vi "Copy to Matching Items.vi"(9 "Front Panel Controls":T1, 11 "VI Data":T2[](array[typedef])) -> (3 "VI Data out":T2[](array[typedef]))   [LabVIEW 2023, in "VI Properties Editor.lvlib"]
doc: "Copies current VI properties to all VIs whose name matches the one currently being edited."
uses:
  VI Properties Editor.lvlib
  <vilib>/picture/picture.llb/imagedata.ctl
  CTLs/VI Data.ctl
  CTLs/VI Properties.ctl
  CTLs/Control Properties.ctl
  CTLs/Main Front Panel Controls.ctl
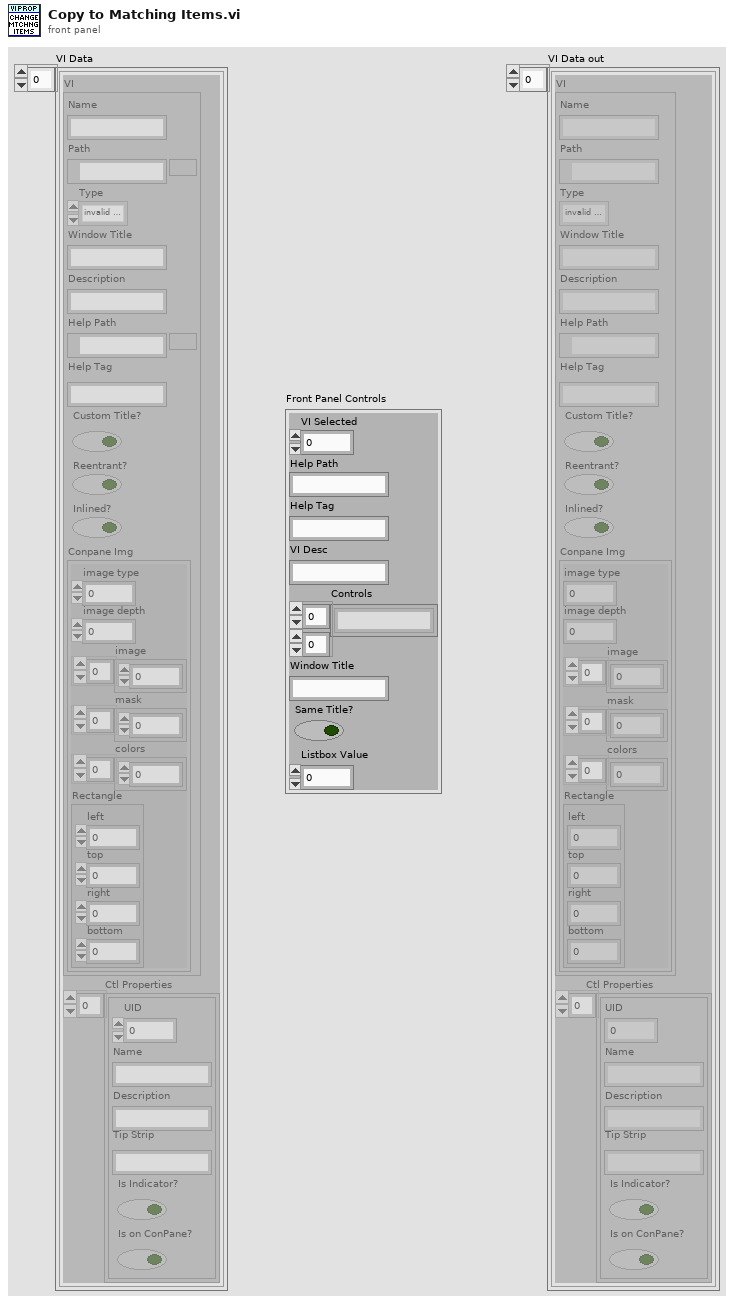
[diagram p1: front panel]
types:
  T1 = typedef "VI Properties Editor.lvlib/Main Front Panel Controls.ctl" = cluster{"VI Selected":i32, "Help Path":string, "Help Tag":string, "VI Desc":string, "Controls":string[][], "Window Title":string, "Same Title?":bool, "Listbox Value":i32}
  T2 = typedef "VI Properties Editor.lvlib/VI Data.ctl" = cluster{"VI":T3, "Ctl Properties":T5[]}
  T3 = typedef "VI Properties Editor.lvlib/VI Properties.ctl" = cluster{"Name":string, "Path":path, "Type":enum32{"invalid VI type", "Standard VI", "Control VI", "Global VI", "Polymorphic VI", "Configuration VI", "SubSystem", "Facade VI", "Method VI", "Statechart Diagram VI"}, "Window Title":string, "Description":string, "Help Path":path, "Help Tag":string, "Custom Title?":bool, "Reentrant?":bool, "Inlined?":bool, "Conpane Img":T4}
  T4 = typedef "imagedata.ctl" = cluster{"image type":i32, "image depth":i32, "image":u8[], "mask":u8[], "colors":u32[], "Rectangle":cluster{"left":i16, "top":i16, "right":i16, "bottom":i16}}
  T5 = typedef "VI Properties Editor.lvlib/Control Properties.ctl" = cluster{"UID":i32, "Name":string, "Description":string, "Tip Strip":string, "Is Indicator?":bool, "Is on ConPane?":bool}
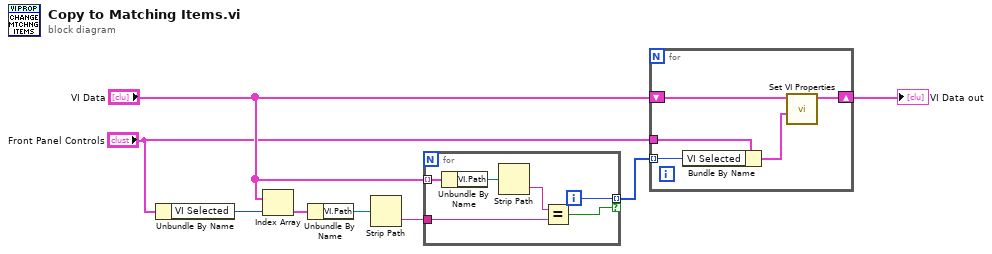
[diagram p0: block diagram]
diagram:
  n1 = Unbundle By Name("Front Panel Controls") -> ("VI Selected"=w4:i32)
  n2 = Index Array(array="VI Data", index=w4) -> (element=w6:T2)
  n3 = Unbundle By Name(w6) -> ("VI.Path"=w3:path)
  n4 = Strip Path(path=w3) -> (name=w2:string)  [unwired: 1 out]
  n5 = for {
    tunnel: "VI Data" -> [w10] mode=indexing
    tunnel: w2 -> [w14]
    tunnel: [w12] -> w7 mode=indexing if=w11
    i -> [w12]
    n6 = Unbundle By Name(w10) -> ("VI.Path"=w9:path)
    n7 = Strip Path(path=w9) -> (name=w13:string)  [unwired: 1 out]
    n8 = Equal?(x=w13, y=w14) -> (x = y?=w11:bool)
  }
  n9 = for {
    tunnel: w7 -> [w16] mode=indexing
    shift-right: [w15] -> w8
    shift-left: "VI Data" -> [w19]
    tunnel: "Front Panel Controls" -> [w18]
    n10 = Bundle By Name(cluster=w18, "VI Selected"=w16) -> (w17:T1)
    n11 = call "Set VI Properties.vi"("Front Panel Controls"=w17, "VI Data"=w19) -> ("VI Data out"=w15:T2[])  [unwired: 9 in]
  }
  "VI Data out" <- w8
